vi "Day 9 Task 2.vi"() -> ()   [LabVIEW 2018]
panel:
  out "product":i32
  out "Array 2":cluster{"row index":i32, "col index":i32}[](array[cluster])
  out "Array":i32[](array[numeric])
  out "output array":i32[](array[numeric])
  out "not 9s = basins":bool[][](array[boolean])
  out "9s":bool[][](array[boolean])
  out "chop out extra edges":bool[][](array[boolean])
  out "appended array":i32[][](array[numeric])
  out "logical AND":bool
  out "Original Array":i32[][](array[numeric])
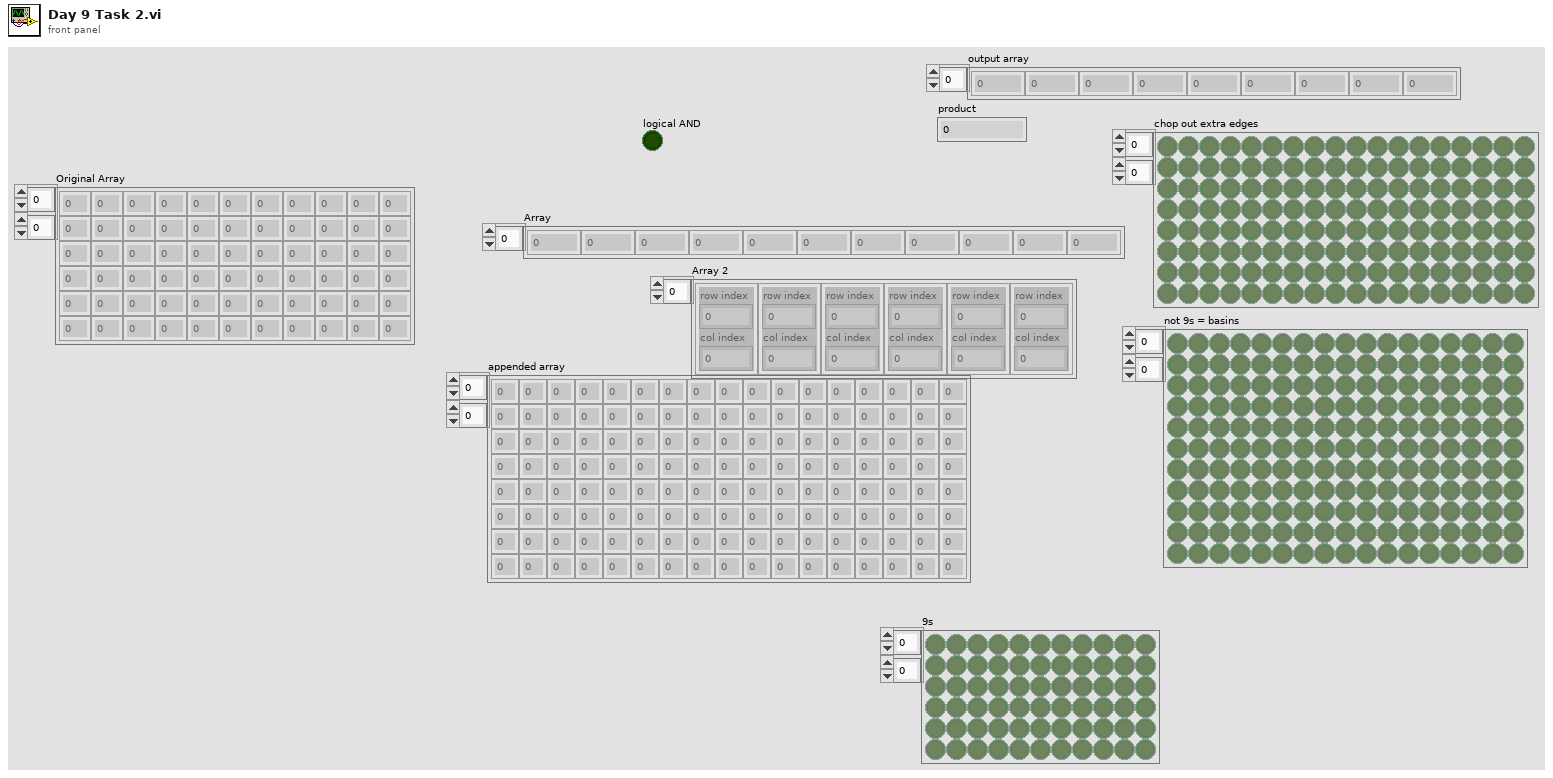
[diagram p1: front panel]
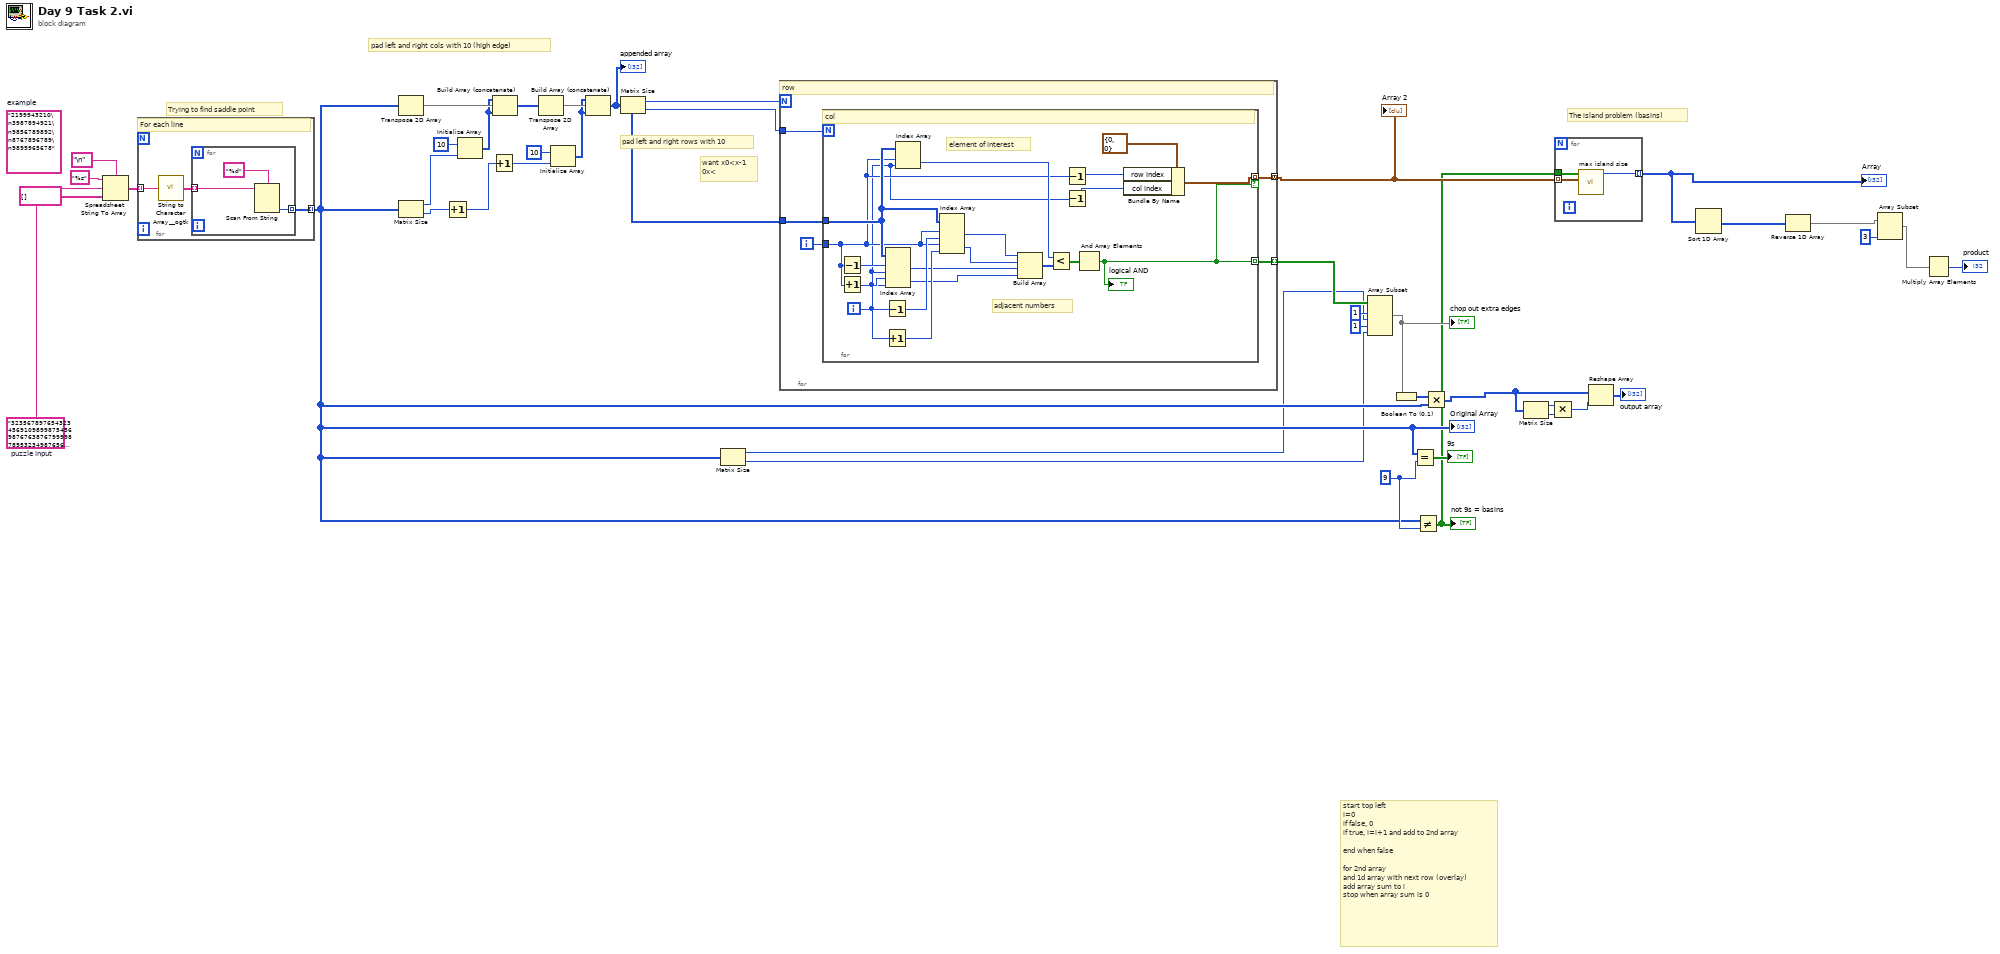
[diagram p0: block diagram]
diagram:
  w18 = 9
  w2 = "3235678976543234569109899875456987676387679999878953234987656895457998743212347892123999912987632489\n2124899989932145698998789994329876545235567899768995349898546789346987654423656789339889899986541678\n1012567897898756797987678989212985432103458987656789456789435691235998775634987897998776798775430567\n2343489956789987976798899578901299654512578998545899567894326890449899896845898945899655987654321378\n3455697645678999875679965467892398999323456789656798998952018921598799987896789235789544398765435459\n45897894325679877645976543586794978789545789969879879995434594336976898999878921234987321298796..."  # puzzle input
  (unwired) "2199943210\n3987894921\n9856789892\n8767896789\n9899965678"  # example
  # "The island problem (basins)"
  # "start top left\ni=0\nif false, 0\nif true, i=i+1 and add to 2nd array\n\nend when false\n\nfor 2nd array\nand 1d array with next row (overlay)\nadd array sum to i\nstop when array sum is 0"
  # "pad left and right rows with 10"
  # "pad left and right cols with 10 (high edge)"
  # "want x0<x-1\n0x<"
  # "Trying to find saddle point"
  n1 = Spreadsheet String To Array(delimiter (Tab)="\n", format string="%s", spreadsheet string=w2, array type (2D Dbl)=string[] []) -> (array=w40:string[])
  n2 = for {
    tunnel: w40 -> [w45] mode=indexing
    tunnel: [w43] -> w17 mode=indexing
    # "For each line"
    n3 = call <userlib>:"String to Character Array__ogtk.vi"("Input String"=w45) -> ("Character Array"=w44:string[])
    n4 = for {
      tunnel: w44 -> [w48] mode=indexing
      tunnel: [w46] -> w43 mode=indexing
      n5 = Scan From String(format string="%d", input string=w48) -> (output 1=w46:i32)  [unwired: 3 in, 3 out]
    }
  }
  "Original Array" <- w17
  n6 = Transpose 2D Array(2D array=w17) -> (transposed array=w38:i32[][])
  n7 = Matrix Size(0:w17) -> (1:w34:i32, 2:w31:i32)
  n8 = Increment(x=w31) -> (x+1=w28:i32)
  n9 = Initialize Array(10 ("element"), w34) -> (w33:i32[])
  n10 = Increment(x=w28) -> (x+1=w30:i32)
  n11 = Build Array (concatenate)(w33, w38, w33) -> (w37:i32[][])
  n12 = Transpose 2D Array(2D array=w37) -> (transposed array=w32:i32[][])
  n13 = Initialize Array(10 ("number of columns"), w30) -> (w29:i32[])
  n14 = Build Array (concatenate)(w29, w32, w29) -> (w23:i32[][])
  "appended array" <- w23
  n15 = Matrix Size(0:w23) -> (1:w26:i32, 2:w27:i32)
  n16 = Matrix Size(0:w17) -> (1:w16:i32, 2:w15:i32)
  n17 = for {
    N: w26 -> [_]
    tunnel: w23 -> [w53]
    tunnel: w27 -> [w52]
    tunnel: [w50] -> w22 mode=indexing
    tunnel: [w49] -> w9 mode=concatenating
    i -> [w51]
    # "row"
    n18 = for {
      N: w52 -> [_]
      tunnel: w53 -> [w68]
      tunnel: w51 -> [w59]
      tunnel: [w60] -> w50 mode=indexing
      tunnel: [w55] -> w49 mode=indexing if=w60
      i -> [w54]
      # "adjacent numbers"
      # "element of interest"
      # "col"
      n19 = Decrement(x=w59) -> (x-1=w67:i32)
      n20 = Increment(x=w59) -> (x+1=w66:i32)
      n21 = Decrement(x=w54) -> (x-1=w72:i32)
      n22 = Increment(x=w54) -> (x+1=w71:i32)
      n23 = Index Array(array=w68, index (row) #1=w67, index (col) #1=w54, index (row) #2=w66, index (col) #2=w54) -> (element #1=w65:i32, element #2=w64:i32)
      n24 = Index Array(array=w68, index (row)=w59, index (col)=w54) -> (element=w63:i32)
      n25 = Index Array(array=w68, index (row) #1=w59, index (col) #1=w72, index (row) #2=w59, index (col) #2=w71) -> (element #1=w70:i32, element #2=w69:i32)
      n26 = Build Array(w70, w69, w65, w64) -> (w62:i32[])
      n27 = Less?(x=w63, y=w62) -> (x < y?=w61:bool[])
      n28 = Decrement(x=w59) -> (x-1=w56:i32)
      n29 = Decrement(x=w54) -> (x-1=w57:i32)
      n30 = And Array Elements(Boolean array=w61) -> (logical AND=w60:bool)
      "logical AND" <- w60
      n31 = Bundle By Name(cluster=cluster{"row index":i32, "col index":i32} {"row index"=0, "col index"=0} ("Coord to check"), "row index"=w56, "col index"=w57) -> (w55:cluster{"row index":i32, "col index":i32})
    }
  }
  "Array 2" <- w9
  n32 = Array Subset(array=w22, index (row)=1 ("index"), length (row)=w16, index (col)=1 ("index"), length (col)=w15) -> (w20:bool[][])
  "chop out extra edges" <- w20
  n33 = Boolean To (0,1)(Boolean=w20) -> (0, 1=w21:i16[][])
  n34 = Equal?(x=w17, y=w18) -> (x = y?=→"9s":bool[][])
  n35 = Not Equal?(x=w17, y=w18) -> (x != y?=w8:bool[][])
  "not 9s = basins" <- w8
  n36 = Multiply(x=w21, y=w17) -> (x*y=w13:i32[][])
  n37 = Matrix Size(0:w13) -> (1:w12:i32, 2:w11:i32)
  n38 = Multiply(x=w12, y=w11) -> (x*y=w10:i32)
  n39 = for {
    tunnel: w9 -> [w75] mode=indexing
    tunnel: w8 -> [w74]
    tunnel: [w73] -> w3 mode=indexing
    n40 = call "max island size.vi"("Coord to check"=w75, "not 9s = basins"=w74) -> ("size of adjacents"=w73:i32)  [unwired: 9 in]
  }
  "Array" <- w3
  n41 = Reshape Array(w13, w10) -> (→"output array":i32[])
  n42 = Sort 1D Array(array=w3) -> (sorted array=w1:i32[])
  n43 = Reverse 1D Array(array=w1) -> (reversed array=w4:i32[])
  n44 = Array Subset(array=w4, length=3) -> (w6:i32[])  [unwired: 1 in]
  n45 = Multiply Array Elements(1:w6) -> (0:→"product":i32)
